vi "Serial Transmitter.vi"(10 "Porta:":refnum<visa-resource-name>, 11 "Robots":T1) -> (0 "error out":errorcluster)   [LabVIEW 2017]
uses:
  <vilib>/Instr/_visa.llb/VISA Configure Serial Port (Instr).vi
  grSim/grSim Robot Command.ctl
panel:
  out "Array":u8[](array[numeric]) format="%02x"
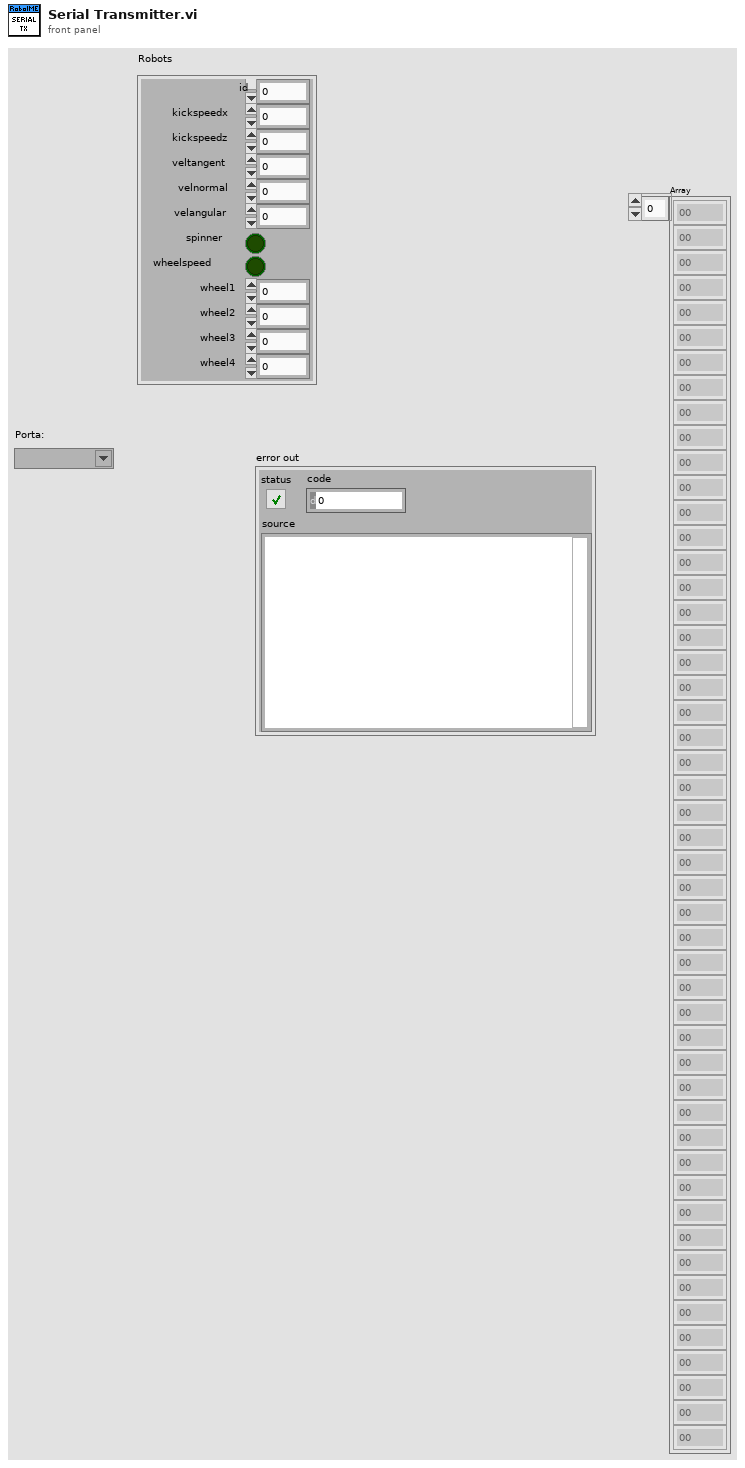
[diagram p1: front panel]
types:
  T1 = typedef "grSim Robot Command.ctl" = cluster{"id":u32, "kickspeedx":sgl, "kickspeedz":sgl, "veltangent":sgl, "velnormal":sgl, "velangular":sgl, "spinner":bool, "wheelspeed":bool, "wheel1":sgl, "wheel2":sgl, "wheel3":sgl, "wheel4":sgl}
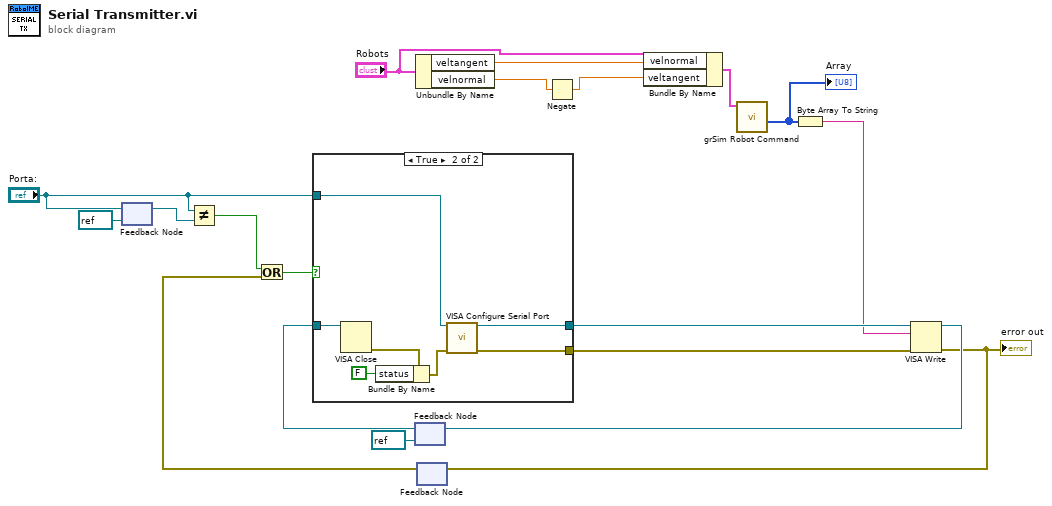
[diagram p0: block diagram]
diagram:
  n1 = feedback #1(refnum<visa-resource-name> refnum ("Porta?")) -> (w19:refnum<visa-resource-name>)
  n2 = feedback-in #1("Porta:") -> ()
  n3 = Not Equal?(x="Porta:", y=w19) -> (x != y?=w8:bool)
  n4 = feedback #2(refnum<visa-resource-name> refnum ("VISA resource name out")) -> (w18:refnum<visa-resource-name>)
  n5 = Unbundle By Name("Robots") -> ("veltangent"=w4:sgl, "velnormal"=w2:sgl)
  n6 = feedback #3() -> (w7:errorcluster)  [unwired: 1 in]
  n7 = Or(x=w8, y=w7) -> (x .or. y?=w9:bool)
  n8 = case shown="True" w9 {
    tunnel: [_ w25] -> w14
    tunnel: [w20 w26] -> w15
    tunnel: "Porta:" -> [_ w21]
    tunnel: w18 -> [w20 w24]
    frame False {
    }
    frame True {
      n9 = VISA Close(VISA resource name=w24) -> (error out=w23:errorcluster)  [unwired: 1 in]
      n10 = Bundle By Name(cluster=w23, "status"=FALSE) -> (w22:errorcluster)
      n11 = call-poly "VISA Configure Serial Port"("VISA resource name"=w21, "error in (no error)"=w22) -> ("VISA resource name out"=w26:refnum<visa-resource-name>, "error out"=w25:errorcluster)  [unwired: 12 in]
    }
  }
  n12 = Negate(x=w2) -> (-x=w1:sgl)
  n13 = Bundle By Name(cluster="Robots", "velnormal"=w4, "veltangent"=w1) -> (w3:T1)
  n14 = call "grSim Robot Command.vi"("Robot"=w3) -> ("Array"=w11:u8[])  [unwired: 10 in]
  "Array" <- w11
  n15 = Byte Array To String(unsigned byte array=w11) -> (string=w13:string)
  n16 = VISA Write(VISA resource name=w15, write buffer=w13, error in (no error)=w14) -> (VISA resource name out=w12:refnum<visa-resource-name>, error out=w10:errorcluster)  [unwired: 1 out]
  "error out" <- w10
  n17 = feedback-in #2(w12) -> ()
  n18 = feedback-in #3(w10) -> ()
